vi "VI Information Change.vi"(8 "error in (no error)":errorcluster, 9 "New":T1[](array[typedef]), 10 "Old":T1[](array[typedef]), 11 "Interface in":refnum<class "Interface.lvclass">) -> (0 "error out":errorcluster, 3 "Interface out":refnum<class "Interface.lvclass">)   [LabVIEW 2015, in "Interface.lvlib" / "Interface.lvclass"]
uses:
  Interface.lvclass
  Interface Messages/VI Information Changed Msg/VI Information Changed Msg.lvclass
  <vilib>/ActorFramework/Actor/Actor.lvclass
  Controls/VI Infomation.ctl
  Interface.lvlib
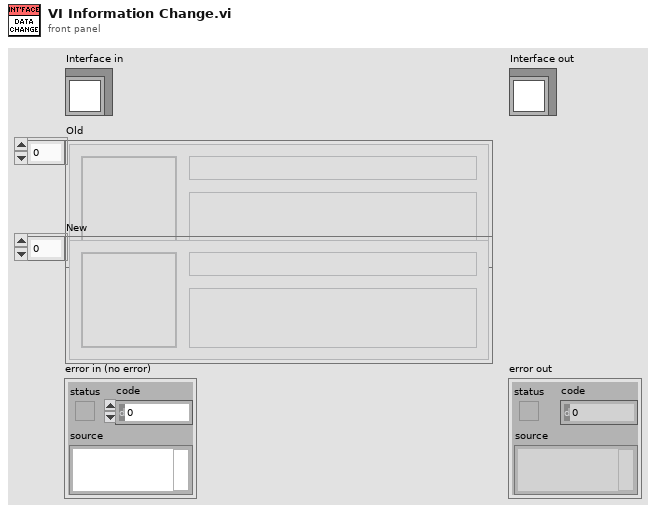
[diagram p1: front panel]
types:
  T1 = typedef "Interface.lvlib/VI Infomation.ctl" = cluster{"VI Name":string, "VI Description":string, "VI Icon":picture}
  T2 = cluster{"VI Name":bool, "VI Description":bool, "VI Icon":bool}[]
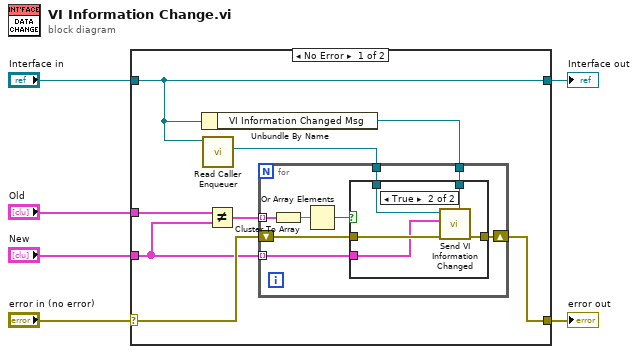
[diagram p0: block diagram]
diagram:
  n1 = case shown="No Error" "error in (no error)" {
    selector: "error in (no error)" -> [w13 w30]
    tunnel: [w14 w30] -> w5
    tunnel: [w12 w29] -> w3
    tunnel: "Interface in" -> [w12 w29]
    tunnel: "Old" -> [w7 _]
    tunnel: "New" -> [w9 _]
    frame No Error {
      n2 = Unbundle By Name(w12) -> ("VI Information Changed Msg"=w8:refnum<class "VI Information Changed Msg.lvclass">)
      n3 = call <vilib>:"Read Caller Enqueuer.vi"("Actor"=w12) -> ("Caller Enqueuer"=w11:refnum<class "Message Enqueuer.lvclass">)  [unwired: 10 in]
      n4 = Not Equal?(x=w7, y=w9) -> (x != y?=w10:T2)
      n5 = for {
        tunnel: w11 -> [w19]
        tunnel: w10 -> [w18] mode=indexing
        tunnel: w9 -> [w17] mode=indexing
        shift-right: [w21] -> w14
        shift-left: w13 -> [w20]
        tunnel: w8 -> [w22]
        n6 = Cluster To Array(cluster=w18) -> (array=w16:bool[])
        n7 = Or Array Elements(Boolean array=w16) -> (logical OR=w15:bool)
        n8 = case shown="True" w15 {
          tunnel: w22 -> [_ w28]
          tunnel: [w23 w27] -> w21
          tunnel: w20 -> [w23 w26]
          tunnel: w19 -> [_ w25]
          tunnel: w17 -> [_ w24]
          frame False {
          }
          frame True {
            n9 = call "Send VI Information Changed.vi"("Message Type"=w28, "error in (no error)"=w26, "VI Infomation"=w24, "Message Enqueuer"=w25) -> ("error out"=w27:errorcluster)  [unwired: 6 in, 1 out]
          }
        }
      }
    }
    frame Error {
    }
  }
  "error out" <- w5
  "Interface out" <- w3
